vi "TestData_MySQL_Inster.vi"(8 "error in (no error)":errorcluster, 9 "data_input":string, 11 "Connection Out":refnum<k7>) -> (0 "error out":errorcluster, 3 "ADODB._Connection Out":refnum<k7>)   [LabVIEW 2012, in "Lib_UEL.ATE.lvlib" / "Lib_TestData.lvlib"]
uses:
  Lib_TestData.lvlib
  App/Lib_App.lvlib
panel:
  out "结果字符串":string
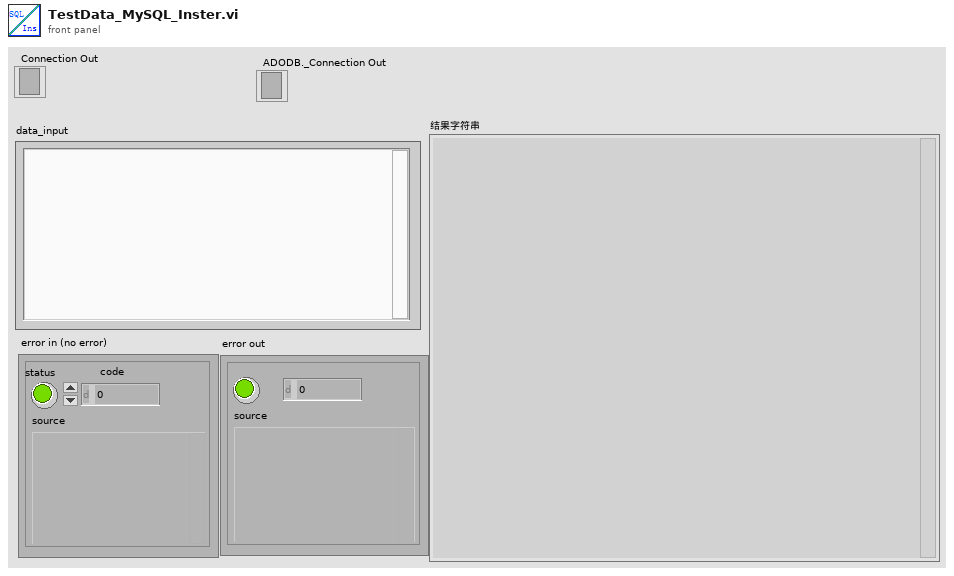
[diagram p1: front panel]
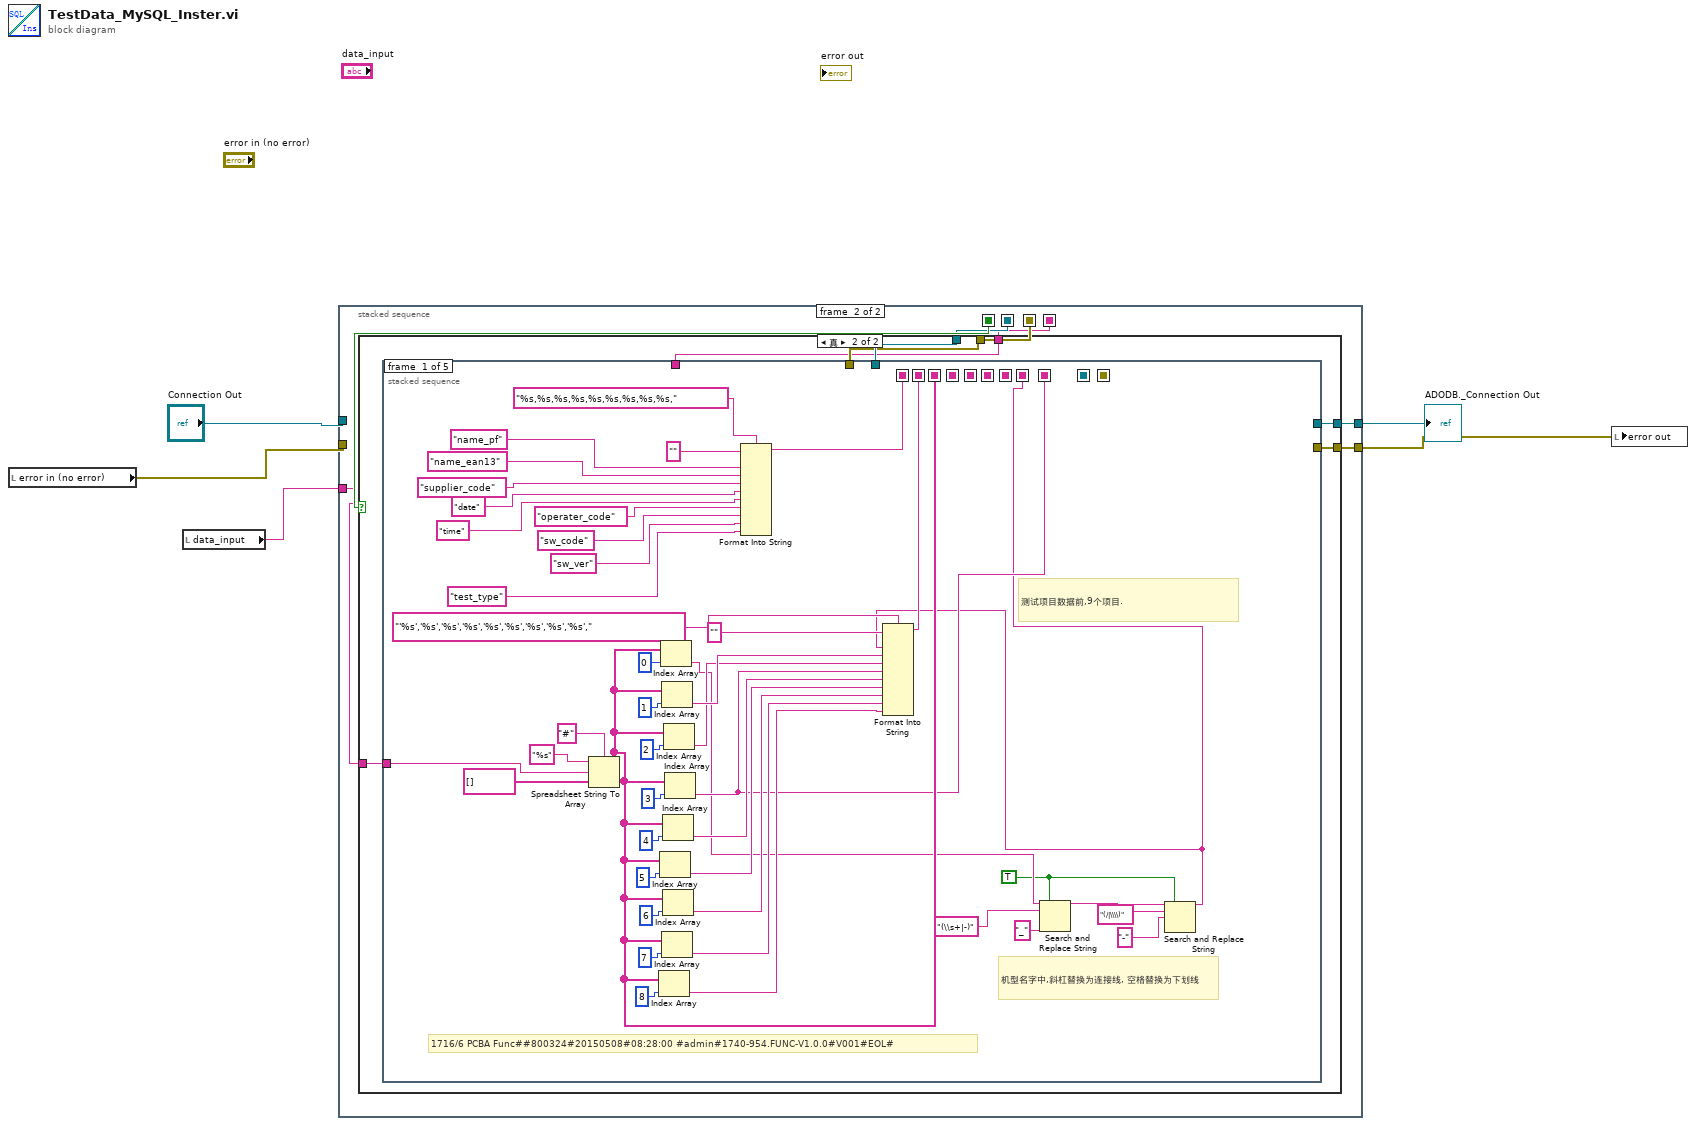
[diagram p0: block diagram]
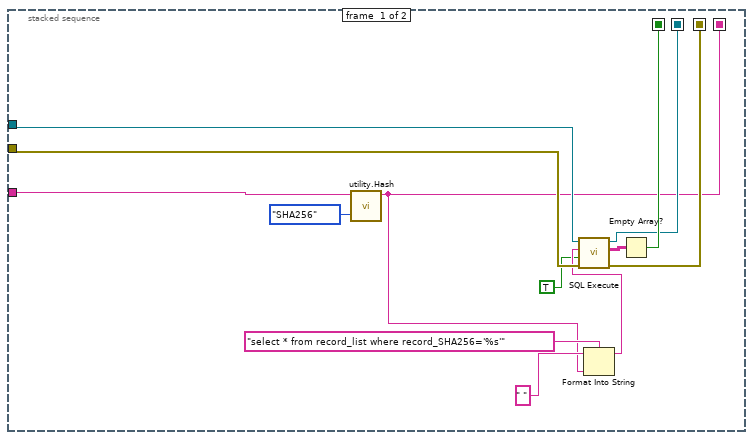
[diagram p2: hidden frame]
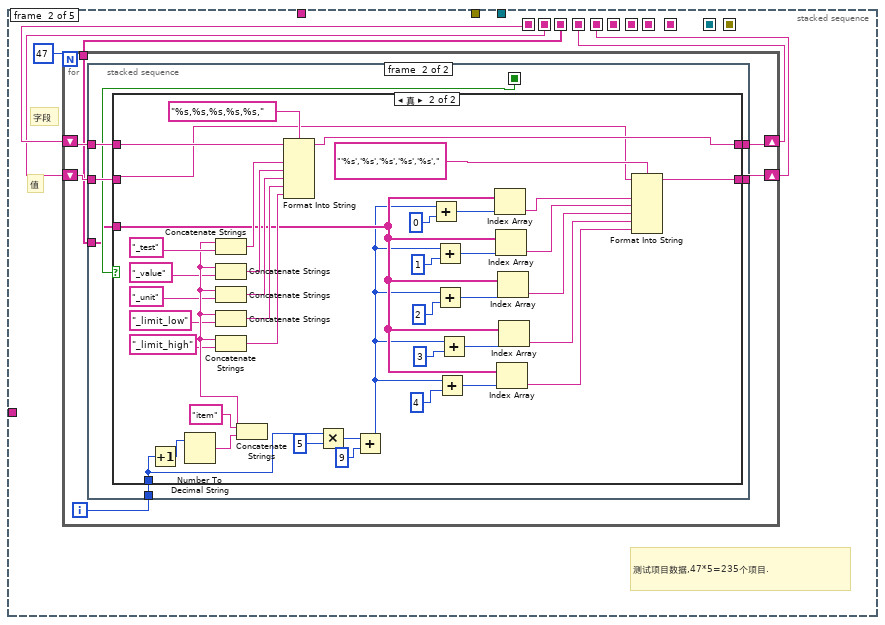
[diagram p4: hidden frame]
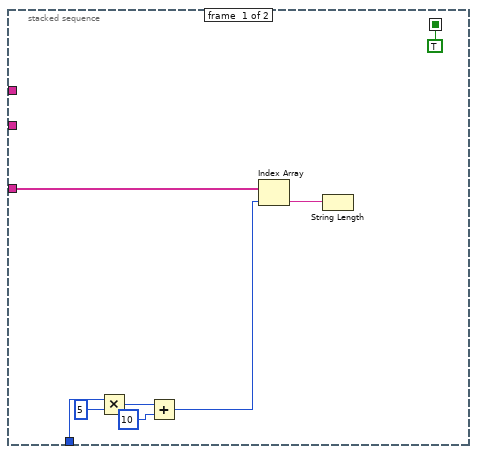
[diagram p5: hidden frame]
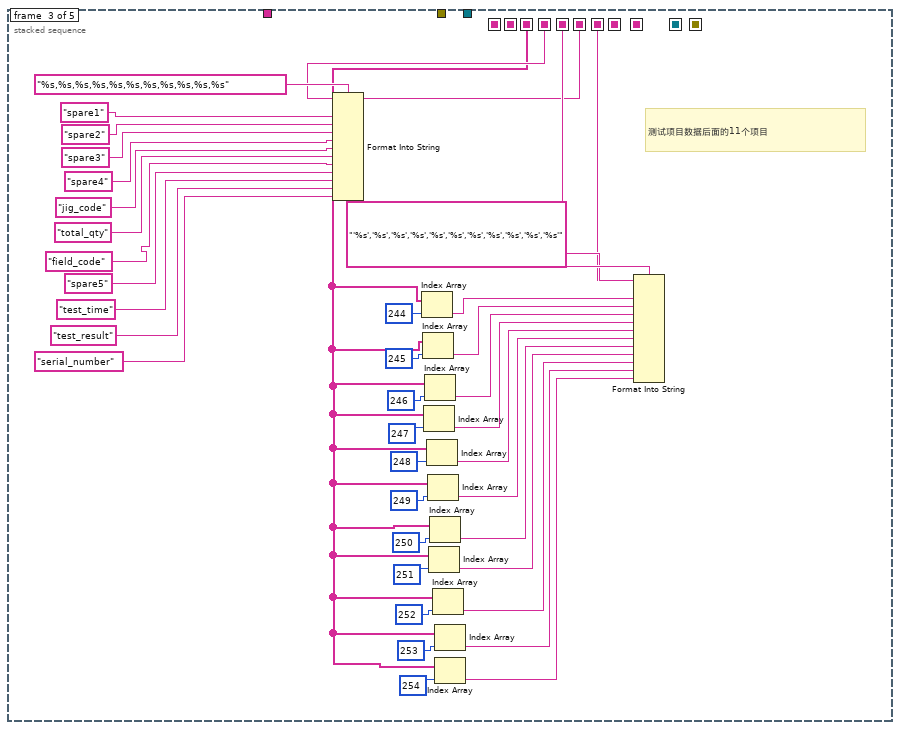
[diagram p7: hidden frame]
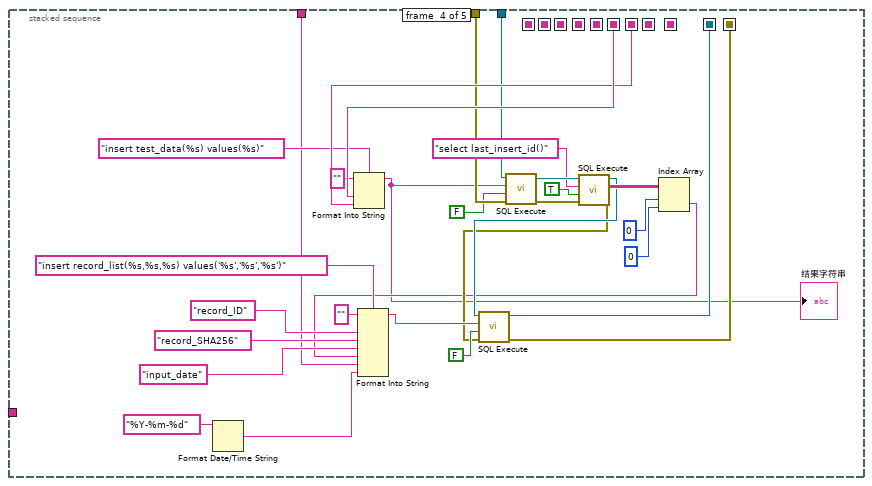
[diagram p8: hidden frame]
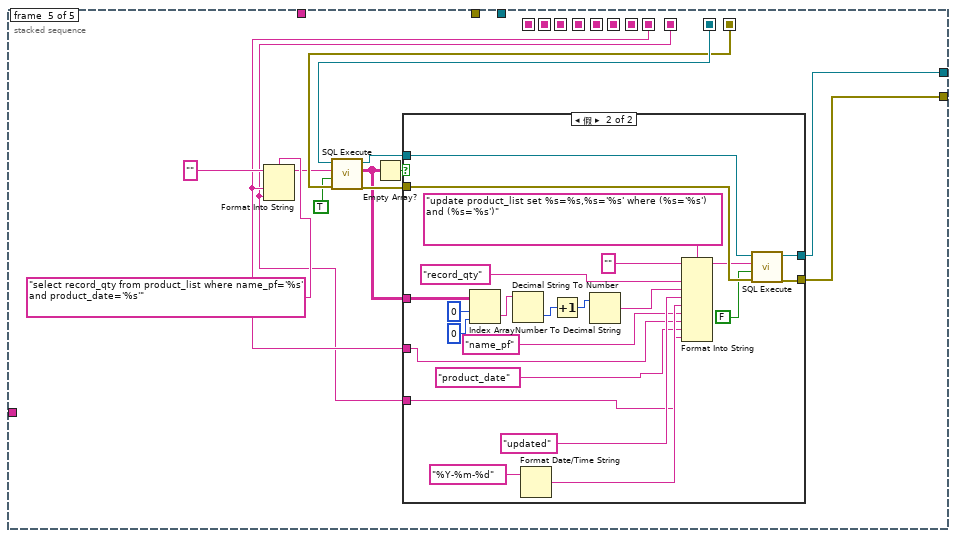
[diagram p9: hidden frame]
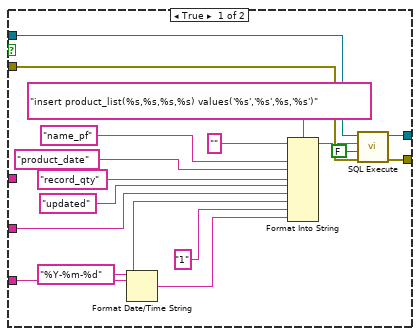
[diagram p10: hidden frame]
diagram:
  n1 = local read "error in (no error)"() -> (w1:errorcluster)
  n2 = local read "data_input"() -> (w3:string)
  n3 = stacked-sequence {
    seq-local: [w15 _] -> [_ w25]
    seq-local: [w9 _] -> [_ w24]
    seq-local: [w8 _] -> [_ w23]
    seq-local: [w7 _] -> [_ w22]
    tunnel: w1 -> [w14 _]
    tunnel: "Connection Out" -> [w10 _]
    tunnel: [_ w21] -> w5
    tunnel: [_ w20] -> w4
    tunnel: w3 -> [w6 w19]
    frame #0 {
      n4 = call "utility.Hash.vi"("Hash_Mode"=enum16{"SHA1", "SHA256", "SHA384", "SHA512"}."SHA256", "Input"=w6) -> ("Hash_Code"=w7:string)  [unwired: 7 in, 2 out]
      n5 = Format Into String(format string="select * from record_list where record_SHA256='%s'" ("格式字符串"), initial string=" " ("字符串"), w7) -> (resulting string=w13:string)  [unwired: 1 in, 1 out]
      n6 = call <userlib>:"SQL Execute.vi"("error in (no error)"=w14, "Return Data (T)"=TRUE, "Command Text"=w13, "ADODB._Connection In"=w10) -> ("error out"=w8:errorcluster, "Data"=w12:string[][], "ADODB._Connection Out"=w9:refnum<k7>)  [unwired: 4 in, 1 out]
      n7 = Empty Array?(array=w12) -> (empty?=w15:bool)
    }
    frame #1 {
      n8 = case shown="真" w25 {
        tunnel: w24 -> [w27 w33]
        tunnel: w23 -> [w26 w32]
        tunnel: w22 -> [_ w31]
        tunnel: [w27 w30] -> w21
        tunnel: [w26 w29] -> w20
        tunnel: w19 -> [_ w28]
        frame False {
        }
        frame True {
          n9 = stacked-sequence {
            seq-local: [w63 _ _ _ _] -> [_ w83 _ _ _]
            seq-local: [w62 _ _ _ _] -> [_ w82 _ _ _]
            seq-local: [w55 _ _ _ _] -> [_ w81 w156 _ _]
            seq-local: [_ w80 _ _ _] -> [_ _ w178 _ _]
            seq-local: [_ w79 _ _ _] -> [_ _ w177 _ _]
            seq-local: [_ _ w175 _ _] -> [_ _ _ w218 _]
            seq-local: [_ _ w176 _ _] -> [_ _ _ w217 _]
            seq-local: [w34 _ _ _ _] -> [_ _ _ _ w226]
            seq-local: [_ _ _ w191 _] -> [_ _ _ _ w232]
            seq-local: [_ _ _ w190 _] -> [_ _ _ _ w231]
            seq-local: [w42 _ _ _ _] -> [_ _ _ _ w219]
            tunnel: w33 -> [_ _ _ w214 _]
            tunnel: w32 -> [_ _ _ w213 _]
            tunnel: w31 -> [_ _ _ w193 _]
            tunnel: [_ _ _ _ w221] -> w30
            tunnel: [_ _ _ _ w220] -> w29
            tunnel: w28 -> [w61 _ _ _ _]
            frame #0 {
              w35 = TRUE
              # "机型名字中,斜杠替换为连接线, 空格替换为下划线"
              # "测试项目数据前,9个项目."
              # "1716/6 PCBA Func##800324#20150508#08:28:00 #admin#1740-954.FUNC-V1.0.0#V001#EOL#"
              n10 = Spreadsheet String To Array(delimiter (Tab)="#" ("分隔符(Tab)"), format string="%s" ("格式字符串"), spreadsheet string=w61, array type (2D Dbl)=string[] []) -> (array=w55:string[])
              n11 = Index Array(array=w55, index=8 ("索引")) -> (element=w51:string)
              n12 = Index Array(array=w55, index=5 ("索引")) -> (element=w54:string)
              n13 = Index Array(array=w55, index=0 ("索引")) -> (element=w36:string)
              n14 = Index Array(array=w55, index=1 ("索引")) -> (element=w68:string)
              n15 = Index Array(array=w55, index=7 ("索引")) -> (element=w52:string)
              n16 = Index Array(array=w55, index=4 ("索引")) -> (element=w64:string)
              n17 = Index Array(array=w55, index=6 ("索引")) -> (element=w53:string)
              n18 = Index Array(array=w55, index=2 ("索引")) -> (element=w57:string)
              n19 = Index Array(array=w55, index=3 ("索引")) -> (element=w42:string)
              n20 = Format Into String(format string="%s,%s,%s,%s,%s,%s,%s,%s,%s," ("格式字符串"), initial string="" ("字符串"), "name_pf" ("输入 1"), "name_ean13" ("输入 1"), "supplier_code" ("输入 1"), "date" ("输入 3"), "time" ("输入 4"), "operater_code" ("输入 1"), "sw_code" ("输入 5"), "sw_ver" ("输入 5"), "test_type" ("输入 5")) -> (resulting string=w63:string)  [unwired: 1 in, 1 out]
              n21 = Search and Replace String(replace all?=w35, input string=w36, search string="(\\s+|-)" ("搜索字符串"), replace string="_" ("替换字符串(\"\")")) -> (result string=w39:string)  [unwired: 4 in, 3 out]
              n22 = Search and Replace String(replace all?=w35, input string=w39, search string="(/|\\\\)" ("替换字符串(\"\")"), replace string="-" ("搜索字符串")) -> (result string=w34:string)  [unwired: 4 in, 3 out]
              n23 = Format Into String(format string="'%s','%s','%s','%s','%s','%s','%s','%s','%s'," ("格式字符串"), initial string="" ("字符串"), w34, w68, w57, w42, w64, w54, w53, w52, w51) -> (resulting string=w62:string)  [unwired: 1 in, 1 out]
            }
            frame #1 {
              # "测试项目数据,47*5=235个项目."
              # "值"
              # "字段"
              n24 = for {
                N: 47 -> [_]
                shift-right: [w88] -> w80
                shift-left: w83 -> [w89]
                shift-right: [w86] -> w79
                shift-left: w82 -> [w87]
                tunnel: w81 -> [w85]
                i -> [w90]
                n25 = stacked-sequence {
                  seq-local: [TRUE _] -> [_ w100]
                  tunnel: w90 -> [w98 w105]
                  tunnel: w89 -> [_ w104]
                  tunnel: [_ w103] -> w88
                  tunnel: w87 -> [_ w102]
                  tunnel: [_ w101] -> w86
                  tunnel: w85 -> [w94 w99]
                  frame #0 {
                    n26 = Multiply(x=w98, y=5) -> (x*y=w96:i32)
                    n27 = Add(x=w96, y=10) -> (x+y=w93:i32)
                    n28 = Index Array(array=w94, index=w93) -> (element=w92:string)
                    n29 = String Length(string=w92) -> ()  [unwired: 1 out]
                  }
                  frame #1 {
                    n30 = case shown="真" w100 {
                      tunnel: w105 -> [_ w131]
                      tunnel: w104 -> [w107 w148]
                      tunnel: [w107 w132] -> w103
                      tunnel: w102 -> [w106 w121]
                      tunnel: [w106 w120] -> w101
                      tunnel: w99 -> [_ w119]
                      frame False {
                      }
                      frame True {
                        n31 = Increment(x=w131) -> (x+1=w146:i32)
                        n32 = Number To Decimal String(number=w146) -> (decimal integer string=w144:string)  [unwired: 1 in]
                        n33 = Concatenate Strings("item", w144) -> (w142:string)
                        n34 = Concatenate Strings(w142, "_test") -> (w137:string)
                        n35 = Concatenate Strings(w142, "_value") -> (w136:string)
                        n36 = Concatenate Strings(w142, "_unit") -> (w135:string)
                        n37 = Concatenate Strings(w142, "_limit_low") -> (w134:string)
                        n38 = Concatenate Strings(w142, "_limit_high") -> (w133:string)
                        n39 = Format Into String(format string="%s,%s,%s,%s,%s," ("格式字符串"), initial string=w148, w137, w136, w135, w134, w133) -> (resulting string=w132:string)  [unwired: 1 in, 1 out]
                        n40 = Multiply(x=w131, y=5) -> (x*y=w129:i32)
                        n41 = Add(x=w129, y=9) -> (x+y=w109:i32)
                        n42 = Add(x=w109, y=0 ("索引")) -> (x+y=w118:i32)
                        n43 = Add(x=w109, y=1 ("索引")) -> (x+y=w115:i32)
                        n44 = Add(x=w109, y=2 ("索引")) -> (x+y=w108:i32)
                        n45 = Add(x=w109, y=4 ("索引")) -> (x+y=w110:i32)
                        n46 = Add(x=w109, y=3 ("索引")) -> (x+y=w112:i32)
                        n47 = Index Array(array=w119, index=w118) -> (element=w126:string)
                        n48 = Index Array(array=w119, index=w115) -> (element=w125:string)
                        n49 = Index Array(array=w119, index=w110) -> (element=w122:string)
                        n50 = Index Array(array=w119, index=w108) -> (element=w124:string)
                        n51 = Index Array(array=w119, index=w112) -> (element=w123:string)
                        n52 = Format Into String(format string="'%s','%s','%s','%s','%s'," ("格式字符串"), initial string=w121, w126, w125, w124, w123, w122) -> (resulting string=w120:string)  [unwired: 1 in, 1 out]
                      }
                    }
                  }
                }
              }
            }
            frame #2 {
              # "测试项目数据后面的11个项目"
              n53 = Format Into String(format string="%s,%s,%s,%s,%s,%s,%s,%s,%s,%s,%s" ("格式字符串"), initial string=w178, "spare1" ("输入 1"), "spare2" ("输入 1"), "spare3" ("输入 1"), "spare4" ("输入 1"), "jig_code" ("输入 1"), "total_qty" ("输入 1"), "field_code" ("输入 1"), "spare5" ("输入 1"), "test_time" ("输入 1"), "test_result" ("输入 3"), "serial_number" ("输入 4")) -> (resulting string=w175:string)  [unwired: 1 in, 1 out]
              n54 = Index Array(array=w156, index=244 ("索引")) -> (element=w185:string)
              n55 = Index Array(array=w156, index=245 ("索引")) -> (element=w183:string)
              n56 = Index Array(array=w156, index=247 ("索引")) -> (element=w179:string)
              n57 = Index Array(array=w156, index=246 ("索引")) -> (element=w180:string)
              n58 = Index Array(array=w156, index=248 ("索引")) -> (element=w155:string)
              n59 = Index Array(array=w156, index=249 ("索引")) -> (element=w154:string)
              n60 = Index Array(array=w156, index=251 ("索引")) -> (element=w152:string)
              n61 = Index Array(array=w156, index=250 ("索引")) -> (element=w153:string)
              n62 = Index Array(array=w156, index=252 ("索引")) -> (element=w151:string)
              n63 = Index Array(array=w156, index=253 ("索引")) -> (element=w150:string)
              n64 = Index Array(array=w156, index=254 ("索引")) -> (element=w149:string)
              n65 = Format Into String(format string="'%s','%s','%s','%s','%s','%s','%s','%s','%s','%s','%s'" ("格式字符串"), initial string=w177, w185, w183, w180, w179, w155, w154, w153, w152, w151, w150, w149) -> (resulting string=w176:string)  [unwired: 1 in, 1 out]
            }
            frame #3 {
              n66 = Format Date/Time String(time format string (%c)="%Y-%m-%d" ("时间格式字符串(%c)")) -> (date/time string=w192:string)  [unwired: 2 in]
              n67 = Format Into String(format string="insert test_data(%s) values(%s)" ("初始字符串"), initial string="" ("初始字符串"), w218, w217) -> (resulting string=w189:string)  [unwired: 1 in, 1 out]
              "结果字符串" <- w189
              n68 = call <userlib>:"SQL Execute.vi"("error in (no error)"=w213, "Return Data (T)"=FALSE, "Command Text"=w189, "ADODB._Connection In"=w214) -> ("error out"=w210:errorcluster, "ADODB._Connection Out"=w211:refnum<k7>)  [unwired: 4 in, 2 out]
              n69 = call <userlib>:"SQL Execute.vi"("error in (no error)"=w210, "Return Data (T)"=TRUE, "Command Text"="select last_insert_id()", "ADODB._Connection In"=w211) -> ("error out"=w197:errorcluster, "Data"=w207:string[][], "ADODB._Connection Out"=w198:refnum<k7>)  [unwired: 4 in, 1 out]
              n70 = Index Array(array=w207, index (row)=0 ("索引 (行)"), index (col)=0 ("禁用的索引 (列)")) -> (element=w194:string)
              n71 = Format Into String(format string="insert record_list(%s,%s,%s) values('%s','%s','%s')" ("初始字符串"), initial string="" ("初始字符串"), "record_ID" ("输入 1"), "record_SHA256" ("输入 1"), "input_date" ("输入 3"), w194, w193, w192) -> (resulting string=w199:string)  [unwired: 1 in, 1 out]
              n72 = call <userlib>:"SQL Execute.vi"("error in (no error)"=w197, "Return Data (T)"=FALSE, "Command Text"=w199, "ADODB._Connection In"=w198) -> ("error out"=w190:errorcluster, "ADODB._Connection Out"=w191:refnum<k7>)  [unwired: 4 in, 2 out]
            }
            frame #4 {
              n73 = Format Into String(format string="select record_qty from product_list where name_pf='%s' and product_date='%s'" ("格式字符串"), initial string="" ("初始字符串"), w226, w219) -> (resulting string=w229:string)  [unwired: 1 in, 1 out]
              n74 = call <userlib>:"SQL Execute.vi"("error in (no error)"=w231, "Return Data (T)"=TRUE, "Command Text"=w229, "ADODB._Connection In"=w232) -> ("error out"=w225:errorcluster, "Data"=w223:string[][], "ADODB._Connection Out"=w224:refnum<k7>)  [unwired: 4 in, 1 out]
              n75 = Empty Array?(array=w223) -> (empty?=w227:bool)
              n76 = case shown="假" w227 {
                tunnel: w226 -> [w236 w258]
                tunnel: w225 -> [w245 w268]
                tunnel: w224 -> [w244 w267]
                tunnel: [w243 w266] -> w221
                tunnel: [w242 w265] -> w220
                tunnel: w223 -> [_ w264]
                tunnel: w219 -> [w235 w251]
                frame True {
                  n77 = Format Date/Time String(time format string (%c)="%Y-%m-%d" ("时间格式字符串(%c)")) -> (date/time string=w233:string)  [unwired: 2 in]
                  n78 = Format Into String(format string="insert product_list(%s,%s,%s,%s) values('%s','%s',%s,'%s')" ("格式字符串"), initial string="" ("初始字符串"), "name_pf" ("输入 1"), "product_date" ("输入 1"), "record_qty" ("输入 1"), "updated" ("输入 1"), w236, w235, "1" ("输入 5"), w233) -> (resulting string=w241:string)  [unwired: 1 in, 1 out]
                  n79 = call <userlib>:"SQL Execute.vi"("error in (no error)"=w245, "Return Data (T)"=FALSE, "Command Text"=w241, "ADODB._Connection In"=w244) -> ("error out"=w242:errorcluster, "ADODB._Connection Out"=w243:refnum<k7>)  [unwired: 4 in, 2 out]
                }
                frame False {
                  n80 = Index Array(array=w264, index (row)=0 ("索引 (行)"), index (col)=0 ("禁用的索引 (列)")) -> (element=w257:string)
                  n81 = Decimal String To Number(string=w257) -> (number=w252:i32)  [unwired: 2 in, 1 out]
                  n82 = Format Date/Time String(time format string (%c)="%Y-%m-%d" ("时间格式字符串(%c)")) -> (date/time string=w260:string)  [unwired: 2 in]
                  n83 = Increment(x=w252) -> (x+1=w256:i32)
                  n84 = Number To Decimal String(number=w256) -> (decimal integer string=w255:string)  [unwired: 1 in]
                  n85 = Format Into String(format string="update product_list set %s=%s,%s='%s' where (%s='%s') and (%s='%s')" ("格式字符串"), initial string="" ("初始字符串"), "record_qty" ("输入 1"), w255, "updated" ("输入 1"), w260, "name_pf" ("输入 5"), w258, "product_date" ("输入 5"), w251) -> (resulting string=w254:string)  [unwired: 1 in, 1 out]
                  n86 = call <userlib>:"SQL Execute.vi"("error in (no error)"=w268, "Return Data (T)"=FALSE, "Command Text"=w254, "ADODB._Connection In"=w267) -> ("error out"=w265:errorcluster, "ADODB._Connection Out"=w266:refnum<k7>)  [unwired: 4 in, 2 out]
                }
              }
            }
          }
        }
      }
    }
  }
  "ADODB._Connection Out" <- w5
  n87 = local write "error out"(w4) -> ()
